vi "扫描.vi"(6 "测试数据":dbl[][](array[numeric]), 7 "XY图":refnum<vi>, 8 "曲线设置":T1={"X轴数据选择"=enum."设置电压", "Y轴组"=[]}, 10 "错误输入（无错误）":errorcluster, 11 "保留数量":i32) -> (2 "错误输出":errorcluster, 3 "突变电压":dbl)   [LabVIEW 2021]
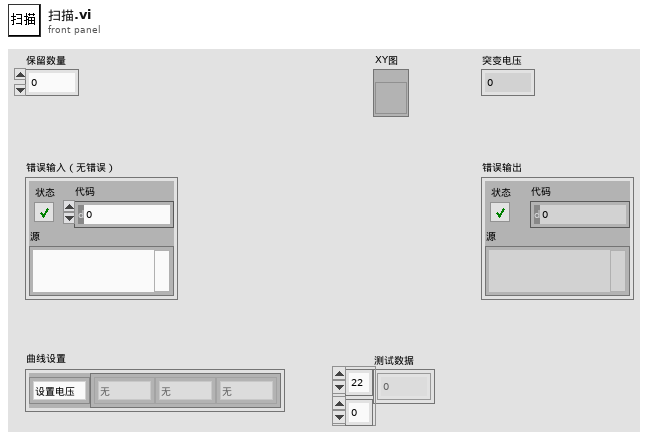
[diagram p1: front panel]
types:
  T1 = typedef "曲线设置.ctl" = cluster{"X轴数据选择":enum16{"时间", "设置电压", "读取电流", "读取电压"}, "Y轴组":enum16{"时间", "设置电压", "读取电流", "读取电压", "无"}[]}
  T2 = cluster{"Name":string, "Color":u32, "Style":u8, "Point Style":u8, "Name Visible":bool, "Allow Drag":bool, "Cursor Mode":u32, "Plot":i32, "Index":i32, "Position":cluster{"X":dbl, "Y":dbl}, "X Scale":u32, "Y Scale":u32, "Watch Plots":i32[], "Watch All Plots":bool, "Plot Area":i32, "Label Offset":cluster{"X":i32, "Y":i32}}
  T3 = cluster{"Name":string, "Color":u32, "Style":u8, "Point Style":u8, "Name Visible":bool, "Allow Drag":bool, "Cursor Mode":u32, "Plot":i32, "Index":i32, "Position":cluster{"X":dbl, "Y":dbl}, "X Scale":u32, "Y Scale":u32, "Watch Plots":i32[], "Watch All Plots":bool, "Plot Area":i32, "Label Offset":cluster{"X":i32, "Y":i32}}[]
  T4 = typedef "曲线属性.ctl" = cluster{"曲线名":string, "曲线颜色":u32}
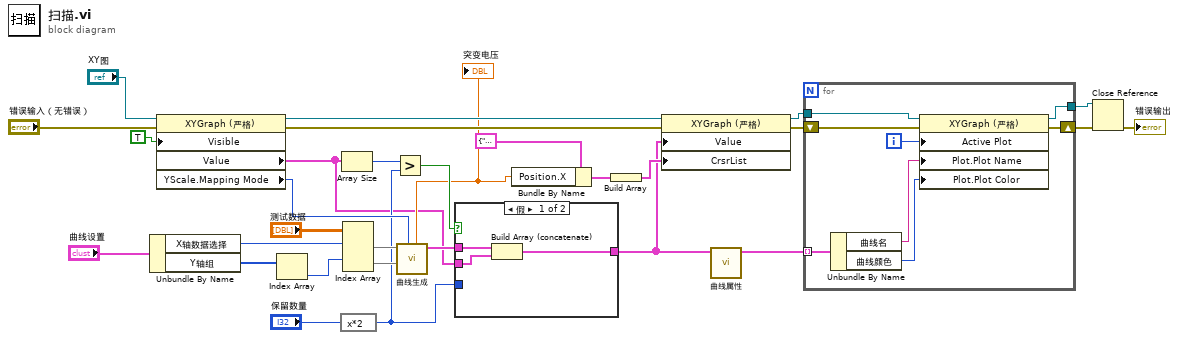
[diagram p0: block diagram]
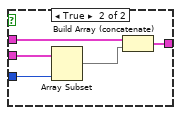
[diagram p2: hidden frame]
diagram:
  n1 = Unbundle By Name("曲线设置") -> ("X轴数据选择"=w29:enum16{"时间", "设置电压", "读取电流", "读取电压"}, "Y轴组"=w28:enum16{"时间", "设置电压", "读取电流", "读取电压", "无"}[])
  n2 = property class="XYGraph (严格)"(reference="XY图", error in="错误输入（无错误）", "Visible"=TRUE ("可见")) -> (reference out=w22:refnum<vi>, error out=w21:errorcluster, "Value"=w3:cluster{"测试数据":dbl[], "测试数据":dbl[]}[], "YScale.Mapping Mode"=w9:u8)
  n3 = Index Array(array=w28) -> (element=w30:enum16{"时间", "设置电压", "读取电流", "读取电压", "无"})  [unwired: 1 in]
  n4 = expression code="x*2"("保留数量") -> (w5:i32)
  n5 = Array Size(array=w3) -> (size(s)=w14:i32)
  n6 = Index Array(array="测试数据", index (row) #1=w29, index (row) #2=w30) -> (element #1=w10:dbl[], element #2=w27:dbl[])  [unwired: 2 in]
  n7 = Greater?(x=w14, y=w5) -> (0:w15:bool)
  n8 = call "曲线生成.vi"("YScale.Mapping Mode"=w9, "Y"=w27, "X"=w10) -> ("曲线"=w7:cluster{dbl[], dbl[]}[], "突变电压"=w8:dbl)  [unwired: 7 in]
  "突变电压" <- w8
  n9 = case shown="假" w15 {
    tunnel: w3 -> [w32 w38]
    tunnel: [w33 w37] -> w1
    tunnel: w5 -> [_ w34]
    tunnel: w7 -> [w31 w35]
    frame False {
      n10 = Build Array (concatenate)(w31, w32) -> (w33:cluster{"测试数据":dbl[], "测试数据":dbl[]}[])
    }
    frame True {
      n11 = Array Subset(array=w38, length=w34) -> (w36:cluster{"测试数据":dbl[], "测试数据":dbl[]}[])  [unwired: 1 in]
      n12 = Build Array (concatenate)(w35, w36) -> (w37:cluster{"测试数据":dbl[], "测试数据":dbl[]}[])
    }
  }
  n13 = Bundle By Name(cluster=T2 {"Name"="游标", "Color"=16776960, "Style"=2, "Point Style"=13, "Name Visible"=FALSE, "Allow Drag"=TRUE, "Cursor Mode"=2, "Plot"=-1, "Index"=0, "Position"={"X"=0.0, "Y"=0.0}, "X Scale"=0, "Y Scale"=0, "Watch Plots"=[], "Watch All Plots"=TRUE, "Plot Area"=0, "Label Offset"={"X"=0, "Y"=0}}, "Position.X"=w8) -> (w11:T2)
  n14 = Build Array(w11) -> (w4:T3)
  n15 = property class="XYGraph (严格)"(reference=w22, error in=w21, "Value"=w1, "CrsrList"=w4) -> (reference out=w20:refnum<vi>, error out=w19:errorcluster)
  n16 = call "曲线属性.vi"("曲线"=w1) -> ("曲线属性"=w13:T4[])  [unwired: 10 in]
  n17 = for {
    shift-right: [w45] -> w18
    shift-left: w19 -> [w46]
    tunnel: w13 -> [w39] mode=indexing
    tunnel: w20 -> [w44]
    tunnel: [w43] -> w17
    i -> [w42]
    n18 = Unbundle By Name(w39) -> ("曲线名"=w41:string, "曲线颜色"=w40:u32)
    n19 = property on="属性节点" class="XYGraph (严格)"(reference=w44, error in=w46, "Active Plot"=w42, "Plot.Plot Name"=w41, "Plot.Plot Color"=w40) -> (reference out=w43:refnum<vi>, error out=w45:errorcluster)
  }
  n20 = Close Reference(reference=w17, error in (no error)=w18) -> (error out=→"错误输出":errorcluster)
